vi "Output to Array.vi"() -> ()   [LabVIEW 2020]
uses:
  3ca1c7ef-2114-4f16-9f2c-0131962597c7.vi
panel:
  in  "Table Control":string[][](table)
  in  "format string":string
  in  "String":string
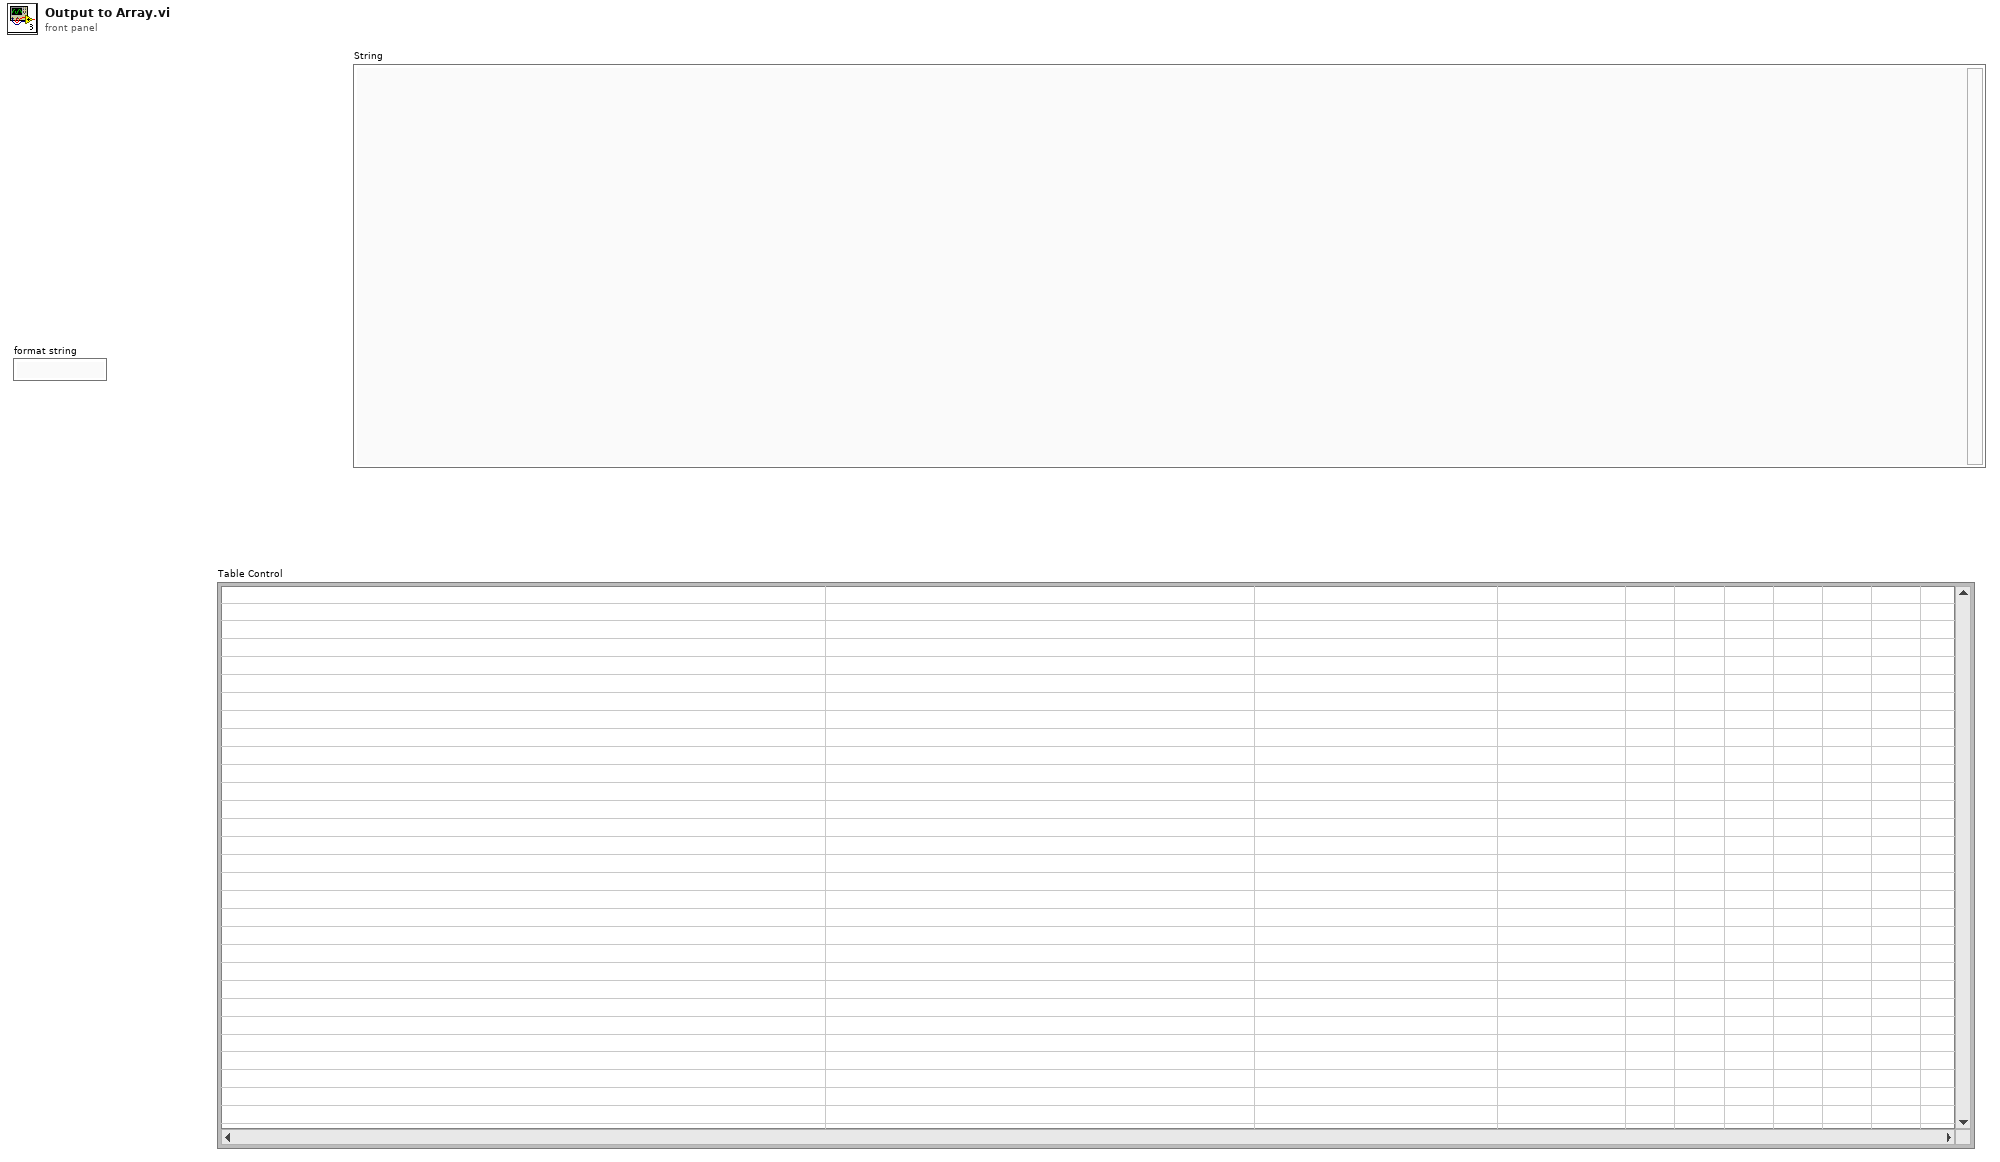
[diagram p1: front panel]
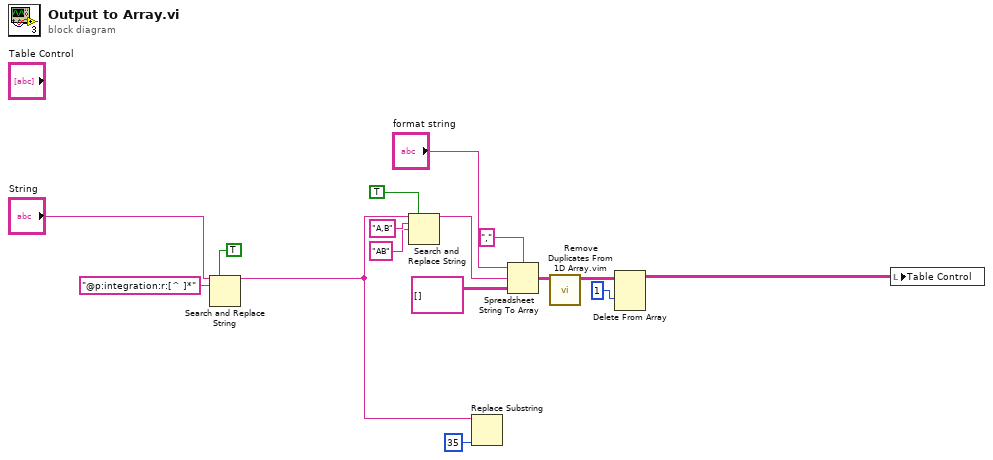
[diagram p0: block diagram]
diagram:
  n1 = Search and Replace String(replace all?=TRUE ("replace all? (F)"), input string="String", search string="@p:integration:r:[^ ]*") -> (result string=w1:string)  [unwired: 5 in, 3 out]
  n2 = Search and Replace String(replace all?=TRUE ("replace all? (F)"), input string=w1, search string="A,B" ("substring (\"\")"), replace string="AB" ("replace string (\"\")")) -> (result string=w6:string)  [unwired: 4 in, 3 out]
  n3 = Replace Substring(2:35 ("length (len. of substring)"), 5:w1) -> ()  [unwired: 2 in, 2 out]
  n4 = Spreadsheet String To Array(delimiter (Tab)=",", format string="format string", spreadsheet string=w6, array type (2D Dbl)=string[][] []) -> (array=w13:string[][])
  n5 = call "Remove Duplicates From 1D Array.vim"("array"=w13) -> ("array with duplicates removed"=w12:string[][])  [unwired: 10 in]
  n6 = Delete From Array(array=w12, index (row)=1) -> (array with subset deleted=w10:string[][])  [unwired: 2 in, 1 out]
  n7 = local write "Table Control"(w10) -> ()
